vi "Fast Move(SubVI for PI).vi"(4 "error in":errorcluster, 5 "Axes":i8, 6 "Milliseconds to wait":u32=20, 7 "Goal Position":dbl=100.0 format="%#_13g") -> (0 "Time of move":u32=101, 1 "error out":errorcluster)   [LabVIEW 2020]
uses:
  Global Parameters.vi
panel:
  out "Position After":dbl[](array[numeric])=[9.994407654, 10.0018692, 6.396408081] format="%.6f"
  in  "USB settings":cluster{"S/N":string, "USB Search?":bool}={"S/N"="0120020544", "USB Search?"=FALSE}
  out "Position Before move":dbl[](array[numeric])=[95.0] format="%.6f"
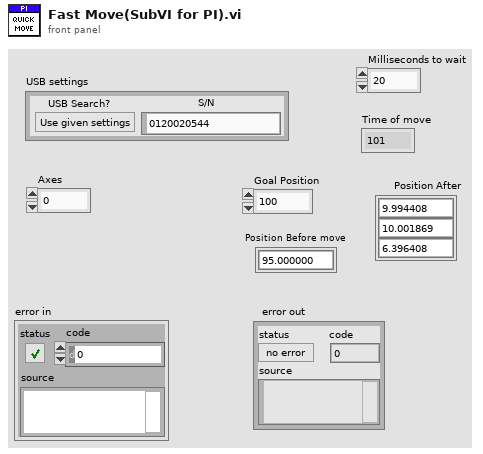
[diagram p1: front panel]
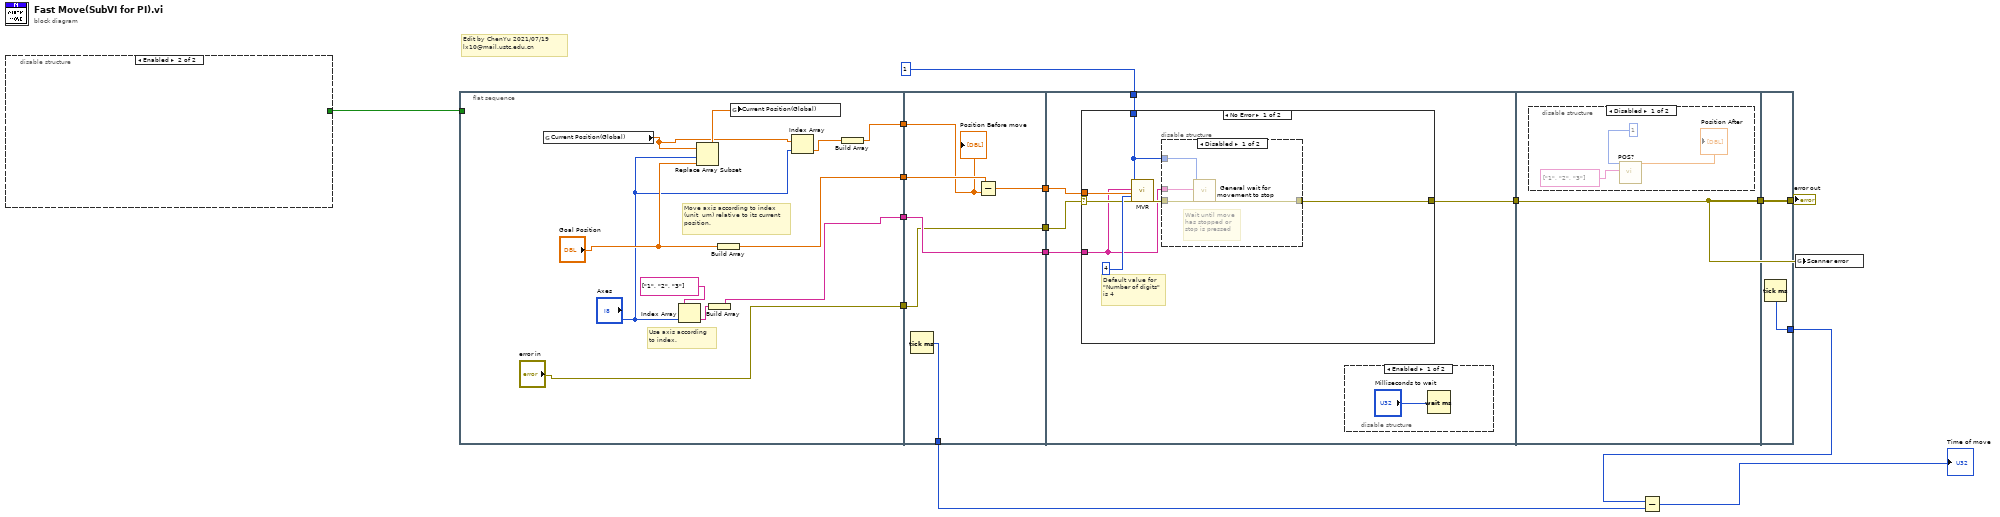
[diagram p0: block diagram]
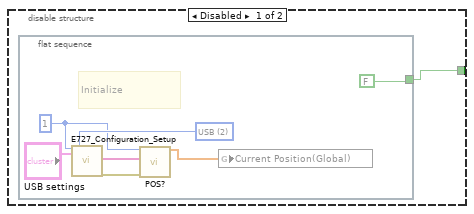
[diagram p2: hidden frame]
diagram:
  # "Edit by ChenYu 2021/07/19 \nlx10@mail.ustc.edu.cn"
  n1 = disable-structure shown="Enabled" {
    disable-tunnel: [w16 _] -> w3
    frame Disabled {
      n2 = flat-sequence {
        tunnel: [FALSE] -> w16
        frame #0 {
          w23 = u16 2 items=["RS232", "TCP/IP", "USB"] ("Interface")
          w22 = 1 ("System no.")
          # "Initialize"
          n3 = call "E727_Configuration_Setup.vi"("System no."=w22, "USB settings"="USB settings", "Interface"=w23) -> ("All conn. axes"=w21:string[], "error out"=w19:errorcluster)  [unwired: 11 in, 4 out]
          n4 = call "POS?.vi"("System no."=w22, "Axes to query"=w21, "error in"=w19) -> ("Position"=w20:dbl[])  [unwired: 2 in, 14 out]
          n5 = global write "Global Parameters.vi" "Current Position(Global)"(w20) -> ()
        }
      }
    }
    frame Enabled {
    }
  }
  n6 = flat-sequence {
    tunnel: w3 -> [_]
    tunnel: ["error in"] -> w7
    tunnel: [w31] -> w6
    tunnel: [w30] -> w5
    tunnel: [w25] -> w4
    tunnel: [w36] -> w15
    tunnel: [w38] -> w14
    tunnel: [w40] -> w13
    tunnel: w7 -> [w36]
    tunnel: w6 -> [w39]
    tunnel: w5 -> [w40]
    tunnel: w4 -> [w37]
    tunnel: [w35] -> w2
    tunnel: 1 -> [w41]
    tunnel: w15 -> [w44]
    tunnel: w14 -> [w43]
    tunnel: w13 -> [w42]
    tunnel: [w45] -> w9
    tunnel: w9 -> [w60]
    tunnel: [w60] -> w1
    tunnel: [w64] -> w8
    tunnel: [w65] -> w11
    tunnel: w1 -> [w65]
    frame #0 {
      # "Use axis according\nto index."
      # "Move axis according to index\n(unit  um) relative to its current\nposition."
      n7 = global read "Global Parameters.vi" "Current Position(Global)"() -> (w28:dbl[])
      n8 = Index Array(array=string[] ["1", "2", "3"], index="Axes") -> (element=w33:string)
      n9 = Replace Array Subset(array=w28, new element="Goal Position", index="Axes") -> (w29:dbl[])
      n10 = Build Array(w33) -> (w30:string[])
      n11 = Build Array("Goal Position") -> (w31:dbl[])
      n12 = global write "Global Parameters.vi" "Current Position(Global)"(w29) -> ()
      n13 = Index Array(array=w28, index="Axes") -> (element=w26:dbl)
      n14 = Build Array(w26) -> (w25:dbl[])
    }
    frame #1 {
      n15 = Tick Count (ms)() -> (millisecond timer value=w35:u32)
      n16 = Subtract(x=w39, y=w37) -> (x-y=w38:dbl[])
      "Position Before move" <- w37
    }
    frame #2 {
      n17 = case shown="No Error" w44 {
        selector: w44 -> [w51 w59]
        tunnel: [w47 w59] -> w45
        tunnel: w41 -> [w48 _]
        tunnel: w43 -> [w50 _]
        tunnel: w42 -> [w49 _]
        frame No Error {
          # "Default value for\n\"Number of digits\"\nis 4"
          n18 = call "MVR.vi"("System no."=w48, "Axes to move"=w49, "Position values"=w50, "No.of digits"=i16 4, "error in"=w51) -> ("error out"=w52:errorcluster)  [unwired: 14 out]
          n19 = disable-structure shown="Disabled" {
            disable-tunnel: w52 -> [w57 w58]
            disable-tunnel: w49 -> [w56 _]
            disable-tunnel: w48 -> [w55 _]
            disable-tunnel: [w54 w58] -> w47
            frame Disabled {
              # "Wait until move\nhas stopped or\nstop is pressed"
              n20 = call "General wait for movement to stop.vi"("System no."=w55, "Axes to wait for"=w56, "error in"=w57) -> ("error out"=w54:errorcluster)  [unwired: 5 in, 11 out]
            }
            frame Enabled {
            }
          }
        }
        frame Error {
          # "Error during initialization"
        }
      }
      n21 = disable-structure shown="Enabled" {
        frame Enabled {
          n22 = Wait (ms)(milliseconds to wait="Milliseconds to wait") -> ()  [unwired: 1 out]
        }
        frame Disabled {
        }
      }
    }
    frame #3 {
      n23 = disable-structure shown="Disabled" {
        frame Disabled {
          n24 = call "POS?.vi"("System no."=1, "Axes to query"=string[] ["1", "2", "3"]) -> ("Position"=→"Position After":dbl[])  [unwired: 3 in, 14 out]
        }
        frame Enabled {
        }
      }
    }
    frame #4 {
      n25 = Tick Count (ms)() -> (millisecond timer value=w64:u32)
    }
  }
  n26 = Subtract(x=w8, y=w2) -> (x-y=→"Time of move":u32)
  n27 = global write "Global Parameters.vi" "Scanner error"(w11) -> ()
  "error out" <- w11
